vi "Read Optical Spectrum.vi"(8 "error in (no error)":errorcluster, 11 "VISA resource name":refnum<visa-resource-name>) -> (0 "error out":errorcluster, 1 "Black Pixel Mean":dbl, 2 "Spectrum by Pixels":dbl[](array[numeric]), 3 "VISA resource name out":refnum<visa-resource-name>)   [LabVIEW 2021, in "Ocean Optics 2000 4000.lvlib"]
doc: "Reads the optical spectra from the spectrometer. The spectrum is displayed in an array according to the pixel number."
uses:
  <instrlib>/Ocean Optics 2000 4000/Ocean Optics 2000 4000.lvlib
  <vilib>/Analysis/baseanly.llb/Mean (DBL).vi
  <vilib>/Analysis/NI_AALBase.lvlib
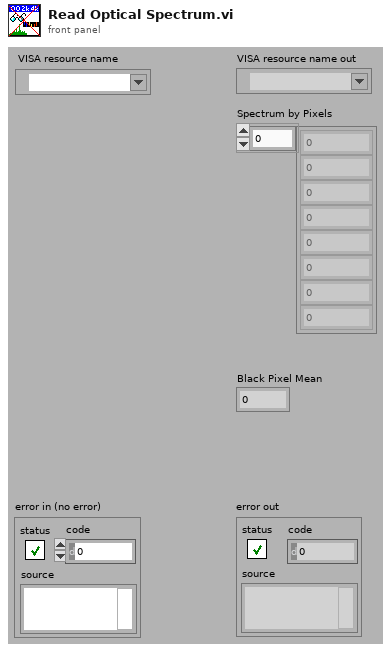
[diagram p1: front panel]
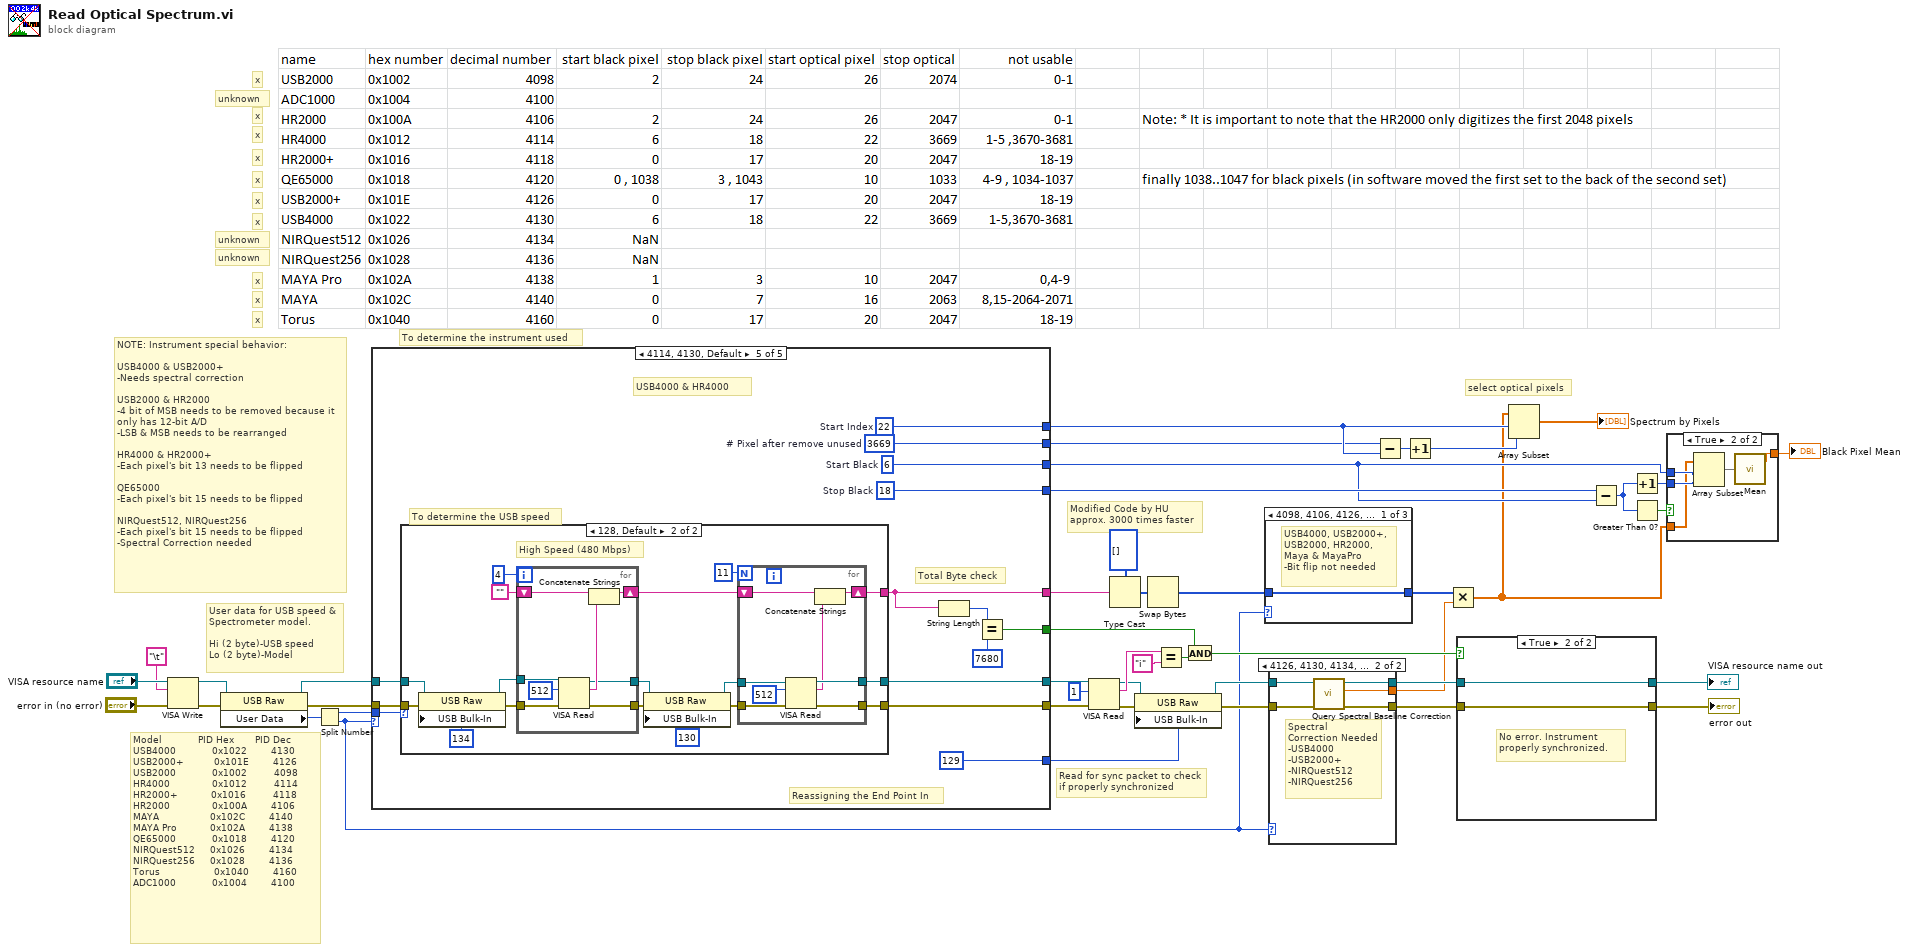
[diagram p0: block diagram]
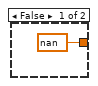
[diagram p2: hidden frame]
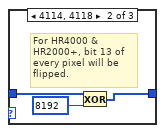
[diagram p3: hidden frame]
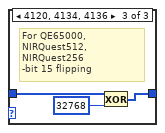
[diagram p4: hidden frame]
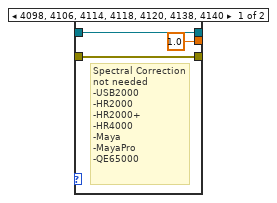
[diagram p5: hidden frame]
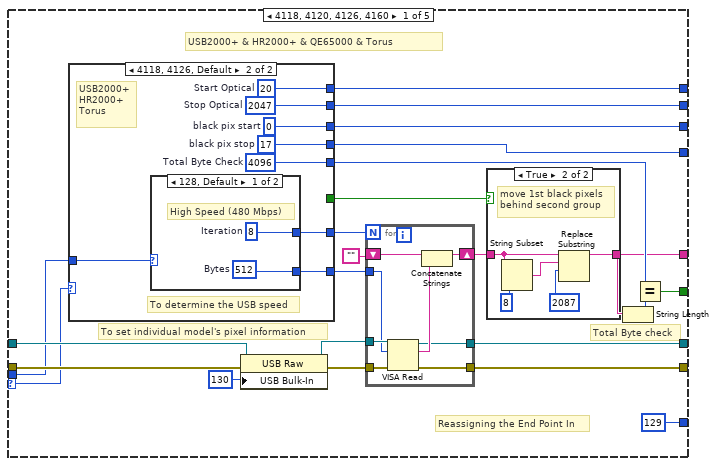
[diagram p6: hidden frame]
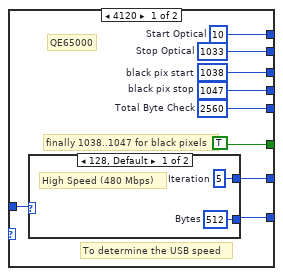
[diagram p8: hidden frame]
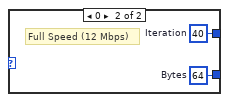
[diagram p9: hidden frame]
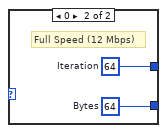
[diagram p10: hidden frame]
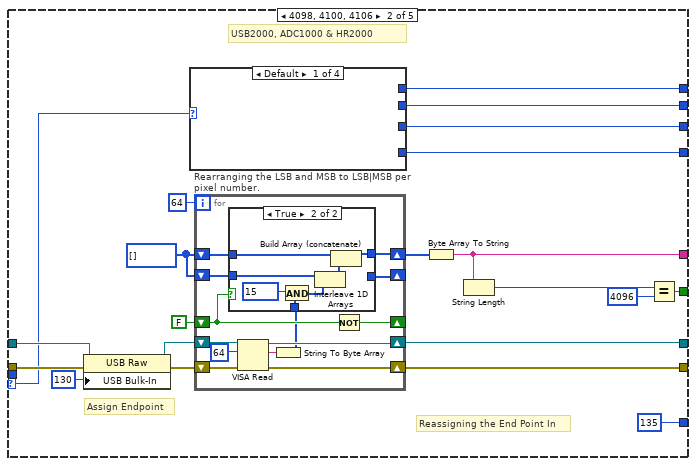
[diagram p11: hidden frame]
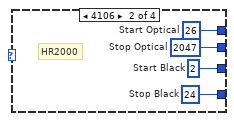
[diagram p12: hidden frame]
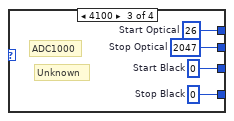
[diagram p13: hidden frame]
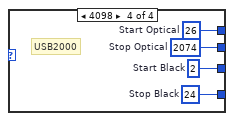
[diagram p14: hidden frame]
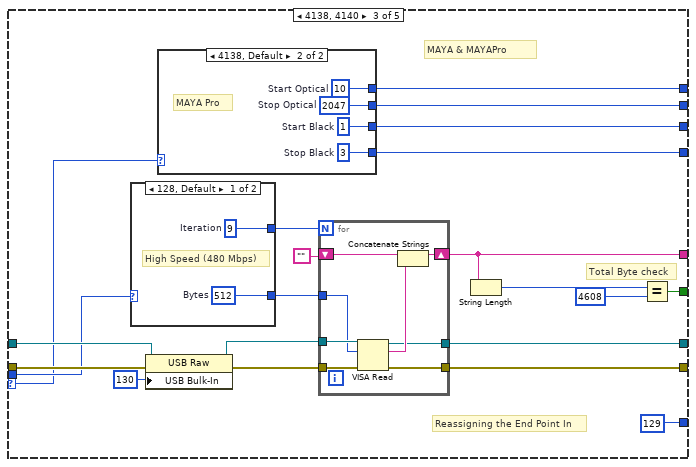
[diagram p16: hidden frame]
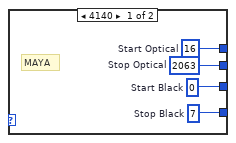
[diagram p17: hidden frame]
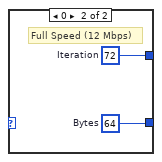
[diagram p18: hidden frame]
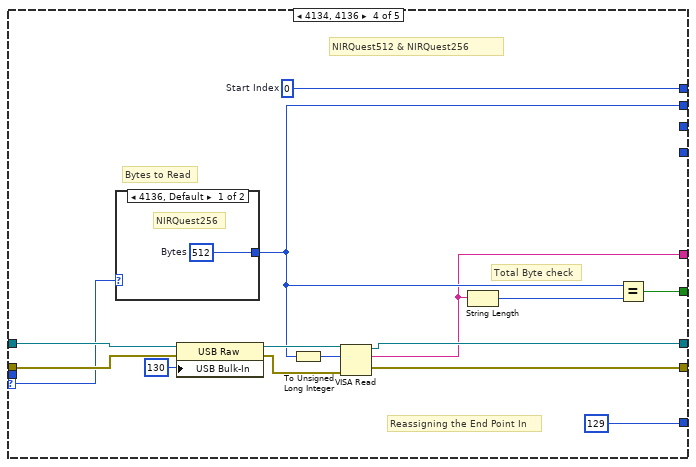
[diagram p19: hidden frame]
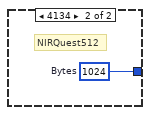
[diagram p20: hidden frame]
diagram:
  # "select optical pixels"
  # "unknown"
  # "unknown"
  # "x"
  # "x"
  # "x"
  # "x"
  # "x"
  # "unknown"
  # "x"
  # "x"
  # "x"
  # "x"
  # "x"
  # "Model            PID Hex       PID Dec \nUSB4000            0x1022        4130 \nUSB2000+          0x101E        4126 \nUSB2000            0x1002         4098\nHR4000              0x1012         4114\nHR2000+           0x1016         4118\nHR2000              0x100A        4106\nMAYA                 0x102C        4140\nMAYA Pro           0x102A        4138\nQE65000            0x1018        4120\nNIRQuest512     0x1026        4134\nNIRQuest256     0x1028        4136\nTorus                  0x1040        4160\nADC1000            0x1004        4100"
  # "Modified Code by HU\napprox. 3000 times faster"
  # "NOTE: Instrument special behavior:\n\nUSB4000 & USB2000+ \n-Needs spectral correction\n\nUSB2000 & HR2000\n-4 bit of MSB needs to be removed because it only has 12-bit A/D\n-LSB & MSB needs to be rearranged \n\nHR4000 & HR2000+\n-Each pixel's bit 13 needs to be flipped\n\nQE65000\n-Each pixel's bit 15 needs to be flipped\n\nNIRQuest512, NIRQuest256\n-Each pixel's bit 15 needs to be flipped\n-Spectral Correction needed"
  # "Read for sync packet to check if properly synchronized"
  # "User data for USB speed & Spectrometer model. \n\nHi (2 byte)-USB speed\nLo (2 byte)-Model"
  # "To determine the instrument used"
  n1 = VISA Write(VISA resource name="VISA resource name", write buffer="\t", error in (no error)="error in (no error)") -> (VISA resource name out=w10:refnum<visa-resource-name>, error out=w42:errorcluster)  [unwired: 1 out]
  n2 = property class="USB Raw"(reference=w10, error in=w42) -> (reference out=w9:refnum<visa-resource-name>, error out=w41:errorcluster, "User Data"=w24:u32)
  n3 = Split Number(x=w24) -> (hi(x)=w23:u16, lo(x)=w15:u16)
  n4 = case shown="4114, 4130, Default" w15 {
    selector: w15 -> [w54 w108 w169 w213 _]
    tunnel: w9 -> [w67 w127 w183 w215 w234]
    tunnel: w41 -> [w68 w126 w182 w214 w233]
    tunnel: [w46 w113 w166 w206 w224] -> w20
    tunnel: [w66 w112 w181 w210 w232] -> w39
    tunnel: [w65 w111 w180 w209 w231] -> w38
    tunnel: [w64 w123 w177 w211 w228] -> w22
    tunnel: w23 -> [w57 _ w172 _ w230]
    tunnel: [w52 w122 w167 w208 w227] -> w3
    tunnel: [w53 w121 w168 w207 w226] -> w6
    tunnel: [i16 129 ("USB Settings:Bulk-In Pipe") i16 135 ("USB Settings:Bulk-In Pipe") i16 129 ("USB Settings:Bulk-In Pipe") i16 129 ("USB Settings:Bulk-In Pipe") i16 129 ("USB Settings:Bulk-In Pipe")] -> w21
    tunnel: [w50 w110 w164 _ w222] -> w13
    tunnel: [w49 w109 w163 _ w221] -> w14
    frame 4118, 4120, 4126, 4160 {
      # "To set individual model's pixel information"
      # "Total Byte check"
      # "Reassigning the End Point In"
      # "USB2000+ & HR2000+ & QE65000 & Torus"
      n5 = case shown="4118, 4126, Default" w54 {
        tunnel: w57 -> [w83 w95]
        tunnel: [w82 w94] -> w56
        tunnel: [w81 w93] -> w55
        tunnel: [w80 w92] -> w53
        tunnel: [w79 w91] -> w52
        tunnel: [w78 w90] -> w51
        tunnel: [w77 w89] -> w50
        tunnel: [w76 w88] -> w49
        tunnel: [TRUE _] -> w48
        frame 4120 {
          w76 = 1047  # black pix stop
          w77 = 1038  # black pix start
          w78 = 2560  # Total Byte Check
          w80 = 10  # Start Optical
          w79 = 1033  # Stop Optical
          # "finally 1038..1047 for black pixels"
          # "To determine the USB speed"
          # "QE65000"
          n6 = case shown="128, Default" w83 {
            tunnel: [w85 w87] -> w82
            tunnel: [w84 w86] -> w81
            frame 128, Default {
              w84 = u32 512  # Bytes
              w85 = 5  # Iteration
              # "High Speed (480 Mbps)"
            }
            frame 0 {
              w86 = u32 64  # Bytes
              w87 = 40  # Iteration
              # "Full Speed (12 Mbps)"
            }
          }
        }
        frame 4118, 4126, Default {
          w88 = 17  # black pix stop
          w89 = 0  # black pix start
          w90 = 4096  # Total Byte Check
          w92 = 20  # Start Optical
          w91 = 2047  # Stop Optical
          # "USB2000+ \nHR2000+\nTorus"
          # "To determine the USB speed"
          n7 = case shown="128, Default" w95 {
            tunnel: [w97 w99] -> w94
            tunnel: [w96 w98] -> w93
            frame 128, Default {
              w96 = u32 512  # Bytes
              w97 = 8  # Iteration
              # "High Speed (480 Mbps)"
            }
            frame 0 {
              w98 = u32 64  # Bytes
              w99 = 64  # Iteration
              # "Full Speed (12 Mbps)"
            }
          }
        }
      }
      n8 = property class="USB Raw"(reference=w67, error in=w68, "USB Bulk-In"=i16 130 ("USB Settings:Bulk-In Pipe")) -> (reference out=w60:refnum<visa-resource-name>, error out=w59:errorcluster)
      n9 = for {
        N: w56 -> [_]
        tunnel: w60 -> [w107]
        tunnel: w59 -> [w106]
        shift-right: [w105] -> w47
        shift-left: "" -> [w104]
        tunnel: [w102] -> w66
        tunnel: [w101] -> w65
        tunnel: w55 -> [w100]
        n10 = VISA Read(VISA resource name=w107, byte count=w100, error in (no error)=w106) -> (VISA resource name out=w102:refnum<visa-resource-name>, read buffer=w103:string, error out=w101:errorcluster)  [unwired: 1 out]
        n11 = Concatenate Strings(w104, w103) -> (w105:string)
      }
      n12 = case shown="True" w48 {
        tunnel: w47 -> [w69 w72]
        tunnel: [w69 w74] -> w46
        frame False {
        }
        frame True {
          # "move 1st black pixels\nbehind second group"
          n13 = String Subset(string=w72, length (rest)=8 ("length (rest)")) -> (substring=w71:string)  [unwired: 1 out]
          n14 = Replace Substring(3:2087 ("offset (0)"), 4:w71, 5:w72) -> (1:w74:string)  [unwired: 2 out]
        }
      }
      n15 = String Length(string=w46) -> (length=w63:i32)
      n16 = Equal?(x=w51, y=w63) -> (x = y?=w64:bool)
    }
    frame 4098, 4100, 4106 {
      w115 = u8[] []
      # "Reassigning the End Point In"
      # "Assign Endpoint"
      # "USB2000, ADC1000 & HR2000"
      n17 = property class="USB Raw"(reference=w127, error in=w126, "USB Bulk-In"=i16 130 ("USB Settings:Bulk-In Pipe")) -> (reference out=w118:refnum<visa-resource-name>, error out=w117:errorcluster)
      n18 = case shown="Default" w108 {
        tunnel: [_ w132 w136 w140] -> w122
        tunnel: [_ w131 w135 w139] -> w121
        tunnel: [_ w130 w134 w138] -> w110
        tunnel: [_ w129 w133 w137] -> w109
        frame Default {
        }
        frame 4106 {
          w130 = 2  # Start Black
          w129 = 24  # Stop Black
          w131 = 26  # Start Optical
          w132 = 2047  # Stop Optical
          # "HR2000"
        }
        frame 4100 {
          w134 = 0  # Start Black
          w133 = 0  # Stop Black
          w135 = 26  # Start Optical
          w136 = 2047  # Stop Optical
          # "Unknown"
          # "ADC1000"
        }
        frame 4098 {
          w138 = 2  # Start Black
          w137 = 24  # Stop Black
          w139 = 26  # Start Optical
          w140 = 2074  # Stop Optical
          # "USB2000"
        }
      }
      n19 = for "Rearranging the LSB and MSB to LSB|MSB per pixel number." {
        N: 64 -> [_]
        shift-right: [w153] -> _
        shift-left: FALSE -> [w152]
        shift-right: [w151] -> _
        shift-left: w115 -> [w150]
        shift-right: [w149] -> w114
        shift-left: w115 -> [w148]
        shift-right: [w143] -> w112
        shift-left: w118 -> [w146]
        shift-right: [w144] -> w111
        shift-left: w117 -> [w145]
        n20 = VISA Read(VISA resource name=w146, byte count=u32 64, error in (no error)=w145) -> (VISA resource name out=w143:refnum<visa-resource-name>, read buffer=w142:string, error out=w144:errorcluster)  [unwired: 1 out]
        n21 = String To Byte Array(string=w142) -> (unsigned byte array=w141:u8[])
        n22 = case shown="True" w152 {
          tunnel: [w154 _] -> w151
          tunnel: w150 -> [_ w162]
          tunnel: [w155 w158] -> w149
          tunnel: w148 -> [w155 w160]
          tunnel: w141 -> [w154 w156]
          frame False {
          }
          frame True {
            n23 = And(x=u8 15, y=w156) -> (x .and. y?=w159:u8[])
            n24 = Interleave 1D Arrays(w162, w159) -> (w161:u8[])
            n25 = Build Array (concatenate)(w160, w161) -> (w158:u8[])
          }
        }
        n26 = Not(x=w152) -> (.not. x?=w153:bool)
      }
      n27 = Byte Array To String(unsigned byte array=w114) -> (string=w113:string)
      n28 = String Length(string=w113) -> (length=w125:i32)
      n29 = Equal?(x=w125, y=4096) -> (x = y?=w123:bool)
    }
    frame 4138, 4140 {
      # "Reassigning the End Point In"
      # "Total Byte check"
      # "MAYA & MAYAPro"
      n30 = case shown="128, Default" w172 {
        tunnel: [w193 w195] -> w171
        tunnel: [w192 w194] -> w170
        frame 128, Default {
          w192 = u32 512  # Bytes
          w193 = 9  # Iteration
          # "High Speed (480 Mbps)"
        }
        frame 0 {
          w194 = u32 64  # Bytes
          w195 = 72  # Iteration
          # "Full Speed (12 Mbps)"
        }
      }
      n31 = property class="USB Raw"(reference=w183, error in=w182, "USB Bulk-In"=i16 130 ("USB Settings:Bulk-In Pipe")) -> (reference out=w175:refnum<visa-resource-name>, error out=w174:errorcluster)
      n32 = case shown="4138, Default" w169 {
        tunnel: [w186 w191] -> w168
        tunnel: [w187 w190] -> w167
        tunnel: [w185 w189] -> w164
        tunnel: [w184 w188] -> w163
        frame 4140 {
          w184 = 7  # Stop Black
          w185 = 0  # Start Black
          w187 = 2063  # Stop Optical
          w186 = 16  # Start Optical
          # "MAYA"
        }
        frame 4138, Default {
          w188 = 3  # Stop Black
          w189 = 1  # Start Black
          w190 = 2047  # Stop Optical
          w191 = 10  # Start Optical
          # "MAYA Pro"
        }
      }
      n33 = for {
        N: w171 -> [_]
        tunnel: w175 -> [w203]
        tunnel: w174 -> [w202]
        shift-right: [w201] -> w166
        shift-left: "" -> [w200]
        tunnel: [w198] -> w181
        tunnel: [w197] -> w180
        tunnel: w170 -> [w196]
        n34 = VISA Read(VISA resource name=w203, byte count=w196, error in (no error)=w202) -> (VISA resource name out=w198:refnum<visa-resource-name>, read buffer=w199:string, error out=w197:errorcluster)  [unwired: 1 out]
        n35 = Concatenate Strings(w200, w199) -> (w201:string)
      }
      n36 = String Length(string=w166) -> (length=w178:i32)
      n37 = Equal?(x=w178, y=4608) -> (x = y?=w177:bool)
    }
    frame 4134, 4136 {
      w207 = 0  # Start Index
      # "Reassigning the End Point In"
      # "Bytes to Read"
      # "Total Byte check"
      # "NIRQuest512 & NIRQuest256"
      n38 = case shown="4136, Default" w213 {
        tunnel: [w219 w220] -> w208
        frame 4136, Default {
          w219 = 512  # Bytes
          # "NIRQuest256"
        }
        frame 4134 {
          w220 = 1024  # Bytes
          # "NIRQuest512"
        }
      }
      n39 = property class="USB Raw"(reference=w215, error in=w214, "USB Bulk-In"=i16 130 ("USB Settings:Bulk-In Pipe")) -> (reference out=w217:refnum<visa-resource-name>, error out=w216:errorcluster)
      n40 = To Unsigned Long Integer(number=w208) -> (unsigned 32bit integer=w204:u32)
      n41 = VISA Read(VISA resource name=w217, byte count=w204, error in (no error)=w216) -> (VISA resource name out=w210:refnum<visa-resource-name>, read buffer=w206:string, error out=w209:errorcluster)  [unwired: 1 out]
      n42 = String Length(string=w206) -> (length=w212:i32)
      n43 = Equal?(x=w208, y=w212) -> (x = y?=w211:bool)
    }
    frame 4114, 4130, Default {
      w221 = 18  # Stop Black
      w222 = 6  # Start Black
      w226 = 22  # Start Index
      w227 = 3669  # # Pixel after remove unused
      # "Reassigning the End Point In"
      # "Total Byte check"
      # "To determine the USB speed"
      # "USB4000 & HR4000"
      n44 = case shown="128, Default" w230 {
        tunnel: w234 -> [w239 w269]
        tunnel: w233 -> [w238 w268]
        tunnel: [w237 w256] -> w232
        tunnel: [w236 w255] -> w231
        tunnel: [w235 w253] -> w224
        frame 0 {
          n45 = property class="USB Raw"(reference=w239, error in=w238, "USB Bulk-In"=i16 130 ("USB Settings:Bulk-In Pipe")) -> (reference out=w243:refnum<visa-resource-name>, error out=w240:errorcluster)
          n46 = for {
            N: 120 -> [_]
            tunnel: w243 -> [w251]
            tunnel: w240 -> [w250]
            tunnel: [w249] -> w237
            tunnel: [w248] -> w236
            shift-right: [w247] -> w235
            shift-left: "" -> [w246]
            # "Full Speed (12 Mbps)"
            n47 = VISA Read(VISA resource name=w251, byte count=u32 64, error in (no error)=w250) -> (VISA resource name out=w249:refnum<visa-resource-name>, read buffer=w245:string, error out=w248:errorcluster)  [unwired: 1 out]
            n48 = Concatenate Strings(w246, w245) -> (w247:string)
          }
        }
        frame 128, Default {
          # "High Speed (480 Mbps)"
          n49 = property class="USB Raw"(reference=w269, error in=w268, "USB Bulk-In"=i16 134 ("USB Settings:Bulk-In Pipe")) -> (reference out=w266:refnum<visa-resource-name>, error out=w265:errorcluster)
          n50 = for {
            N: 4 -> [_]
            tunnel: w266 -> [w277]
            tunnel: w265 -> [w276]
            shift-right: [w270] -> w254
            shift-left: "" -> [w274]
            tunnel: [w272] -> w260
            tunnel: [w271] -> w259
            n51 = VISA Read(VISA resource name=w277, byte count=u32 512, error in (no error)=w276) -> (VISA resource name out=w272:refnum<visa-resource-name>, read buffer=w273:string, error out=w271:errorcluster)  [unwired: 1 out]
            n52 = Concatenate Strings(w274, w273) -> (w270:string)
          }
          n53 = property class="USB Raw"(reference=w260, error in=w259, "USB Bulk-In"=i16 130 ("USB Settings:Bulk-In Pipe")) -> (reference out=w263:refnum<visa-resource-name>, error out=w257:errorcluster)
          n54 = for {
            N: 11 -> [_]
            tunnel: w263 -> [w284]
            tunnel: w257 -> [w283]
            tunnel: [w282] -> w256
            tunnel: [w281] -> w255
            shift-right: [w280] -> w253
            shift-left: w254 -> [w279]
            n55 = VISA Read(VISA resource name=w284, byte count=u32 512, error in (no error)=w283) -> (VISA resource name out=w282:refnum<visa-resource-name>, read buffer=w278:string, error out=w281:errorcluster)  [unwired: 1 out]
            n56 = Concatenate Strings(w279, w278) -> (w280:string)
          }
        }
      }
      n57 = String Length(string=w224) -> (length=w223:i32)
      n58 = Equal?(x=w223, y=7680) -> (x = y?=w228:bool)
    }
  }
  n59 = VISA Read(VISA resource name=w39, byte count=u32 1, error in (no error)=w38) -> (VISA resource name out=w33:refnum<visa-resource-name>, read buffer=w37:string, error out=w32:errorcluster)  [unwired: 1 out]
  n60 = Type Cast(type=u16[] [], x=w20) -> (*(type *) &x=w19:u16[])
  n61 = property class="USB Raw"(reference=w33, error in=w32, "USB Bulk-In"=w21) -> (reference out=w31:refnum<visa-resource-name>, error out=w30:errorcluster)
  n62 = Swap Bytes(anything=w19) -> (byte swapped=w17:u16[])
  n63 = Equal?(x=w37, y="i") -> (x = y?=w34:bool)
  n64 = And(x=w22, y=w34) -> (x .and. y?=w35:bool)
  n65 = case shown="4098, 4106, 4126, 4130, 4138, 4140, Default" w15 {
    tunnel: w17 -> [w286 w289 w291]
    tunnel: [w286 w287 w290] -> w16
    frame 4098, 4106, 4126, 4130, 4138, 4140, Default {
      # "USB4000, USB2000+, USB2000, HR2000, Maya & MayaPro\n-Bit flip not needed"
    }
    frame 4114, 4118 {
      # "For HR4000 & HR2000+, bit 13 of every pixel will be flipped."
      n66 = Exclusive Or(1:u16 8192 ("y"), 2:w289) -> (0:w287:u16[])
    }
    frame 4120, 4134, 4136 {
      # "For QE65000, NIRQuest512, NIRQuest256 \n-bit 15 flipping"
      n67 = Exclusive Or(1:u16 32768 ("y"), 2:w291) -> (0:w290:u16[])
    }
  }
  n68 = case shown="4126, 4130, 4134, 4136, Default" w15 {
    tunnel: w31 -> [w295 w300]
    tunnel: w30 -> [w294 w299]
    tunnel: [w295 w298] -> w29
    tunnel: [w294 w297] -> w28
    tunnel: [1.0 ("Spectral Baseline Correction") w296] -> w25
    frame 4098, 4106, 4114, 4118, 4120, 4138, 4140 {
      # "Spectral Correction not needed\n-USB2000\n-HR2000\n-HR2000+\n-HR4000\n-Maya\n-MayaPro\n-QE65000"
    }
    frame 4126, 4130, 4134, 4136, Default {
      # "Spectral Correction Needed\n-USB4000\n-USB2000+\n-NIRQuest512\n-NIRQuest256"
      n69 = call <instrlib>:"Query Spectral Baseline Correction.vi"("error in (no error)"=w299, "VISA resource name"=w300) -> ("error out"=w297:errorcluster, "Spectral Baseline Correction"=w296:dbl, "VISA resource name out"=w298:refnum<visa-resource-name>)  [unwired: 7 out]
    }
  }
  n70 = Subtract(x=w3, y=w6) -> (x-y=w5:i32)
  n71 = Increment(x=w5) -> (x+1=w4:i32)
  n72 = Multiply(x=w16, y=w25) -> (x*y=w2:dbl[])
  n73 = case shown="True" w35 {
    tunnel: w28 -> [w303 w309]
    tunnel: [w305 w309] -> w26
    tunnel: [w304 w308] -> w27
    tunnel: w29 -> [w304 w308]
    frame False {
      # "Error"
      n74 = call <vilib>:"Error Cluster From Error Code.vi"("error message (\"\")"="Instrument not synchronized properly. Power cycle the instrument." ("error message (\"\")"), "error code (0)"=-1074001919 ("code")) -> ("error out"=w302:errorcluster)  [unwired: 2 in, 5 out]
      n75 = Build Array(w303, w302) -> (w301:errorcluster[])
      n76 = Merge Errors(w301) -> (w305:errorcluster)
    }
    frame True {
      # "No error. Instrument properly synchronized."
    }
  }
  "VISA resource name out" <- w27
  "error out" <- w26
  n77 = Array Subset(array=w2, index=w6, length=w4) -> (→"Spectrum by Pixels":dbl[])
  n78 = Subtract(x=w14, y=w13) -> (x-y=w8:i32)
  n79 = Increment(x=w8) -> (x+1=w7:i32)
  n80 = Greater Than 0?(x=w8) -> (x > 0?=w12:bool)
  n81 = case shown="True" w12 {
    tunnel: w13 -> [_ w315]
    tunnel: w7 -> [_ w314]
    tunnel: [nan ("mean") w312] -> w11
    tunnel: w2 -> [_ w311]
    frame False {
    }
    frame True {
      n82 = Array Subset(array=w311, index=w315, length=w314) -> (w313:dbl[])
      n83 = call-poly <vilib>:"Mean.vi"("X"=w313) -> ("mean"=w312:dbl)  [unwired: 1 out]
    }
  }
  "Black Pixel Mean" <- w11
